vi "Tipo de guardado.vi"(8 "error in (no error)":errorcluster, 10 "Tipo de Guardado":enum16{"Tdms", "Txt"}(ring), 11 "Contador Binario in":refnum<class "Contador Binario.lvclass">) -> (0 "error out":errorcluster, 3 "Contador Binario out":refnum<class "Contador Binario.lvclass">)   [LabVIEW 2020, in "Contador Binario.lvlib" / "Contador Binario.lvclass"]
uses:
  Contador Binario.lvclass
  C:/Program Files (x86)/National Instruments/LabVIEW 2020/vi.lib/ActorFramework/Actor/Actor.lvclass
  Contador Binario.lvclass/Contador Binario.ctl
  Logging Tdms/Logging Tdms/Logging Tdms.lvclass
  C:/Users/Alex/Documents/Tarea-Actor/Logging Txt/Logging Txt/Logging Txt.lvclass
  Logging Txt/Logging Txt/Logging Txt.lvclass
  <vilib>/ActorFramework/Message Enqueuer/Message Enqueuer.lvclass/Message Enqueuer.ctl
  <vilib>/ActorFramework/Message Enqueuer/Enqueue.vi
  <vilib>/ActorFramework/Stop Msg/Stop Msg.lvclass
  C:/Program Files (x86)/National Instruments/LabVIEW 2020/vi.lib/ActorFramework/Message/Message.lvclass
  <vilib>/ActorFramework/Message Priority Queue/Priority Enqueue.vi
  <vilib>/ActorFramework/Actor/Actor.lvclass
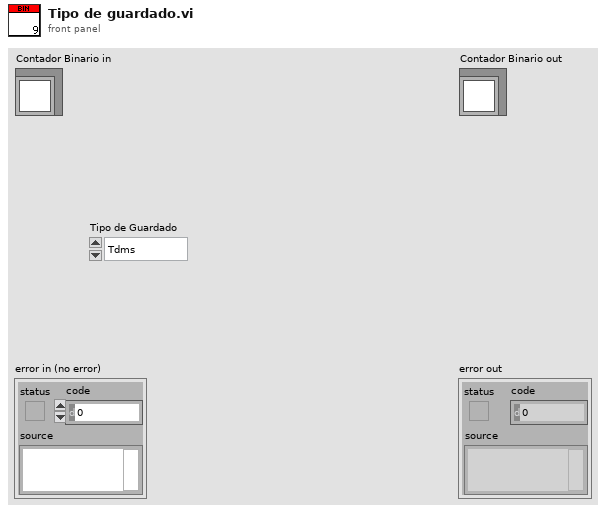
[diagram p1: front panel]
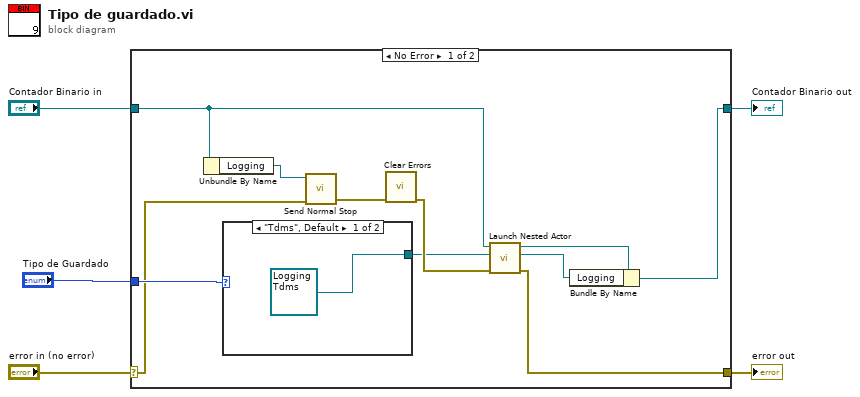
[diagram p0: block diagram]
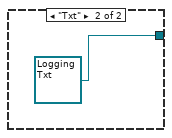
[diagram p2: hidden frame]
diagram:
  n1 = case shown="No Error" "error in (no error)" {
    selector: "error in (no error)" -> [w8 w20]
    tunnel: [w9 w20] -> w4
    tunnel: [w13 w19] -> w2
    tunnel: "Contador Binario in" -> [w15 w19]
    tunnel: "Tipo de Guardado" -> [w16 _]
    frame No Error {
      n2 = Unbundle By Name(w15) -> ("Logging"=w12:refnum<class "Message Enqueuer.lvclass">)
      n3 = case shown="\"Tdms\", Default" w16 {
        tunnel: [refnum<class "Logging Tdms.lvclass"> refnum ("Logging Tdms.lvlib:Logging Tdms.lvclass") refnum<class "Logging Txt.lvclass"> refnum ("Logging Txt.lvlib:Logging Txt.lvclass")] -> w6
        frame "Tdms", Default {
        }
        frame "Txt" {
        }
      }
      n4 = call <vilib>:"Send Normal Stop.vi"("error in (no error)"=w8, "Message Enqueuer"=w12) -> ("error out"=w11:errorcluster)  [unwired: 9 in]
      n5 = call <vilib>:"Clear Errors.vi"("error in (no error)"=w11) -> ("error out"=w10:errorcluster)  [unwired: 5 in, 1 out]
      n6 = call <vilib>:"Launch Nested Actor.vi"("error in (no error)"=w10, "Nested Actor"=w6, "Caller Actor in"=w15) -> ("error out"=w9:errorcluster, "Nested Actor's Enqueuer"=w7:refnum<class "Message Enqueuer.lvclass">, "Caller Actor out"=w14:refnum<class "Contador Binario.lvclass">)  [unwired: 6 in]
      n7 = Bundle By Name(cluster=w14, "Logging"=w7) -> (w13:refnum<class "Contador Binario.lvclass">)
    }
    frame Error {
    }
  }
  "error out" <- w4
  "Contador Binario out" <- w2
